vi "Read Signal Message.vi"(6 "timeout ms (25000)":i32=25000, 8 "error in (no error)":errorcluster, 11 "CLI in":refnum<class "CLI.lvclass">) -> (0 "error out":errorcluster, 1 "Message Contents":string, 2 "Message Type":string, 3 "CLI out":refnum<class "CLI.lvclass">)   [LabVIEW 2017, in "CLI.lvclass"]
uses:
  CLI.lvclass
  CLI.lvclass/CLI.ctl
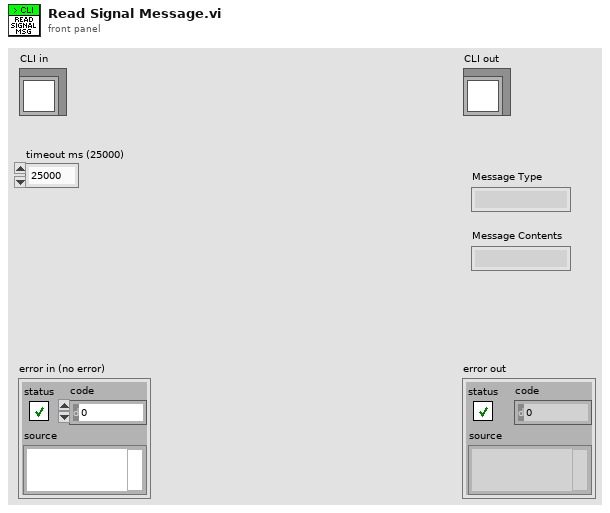
[diagram p1: front panel]
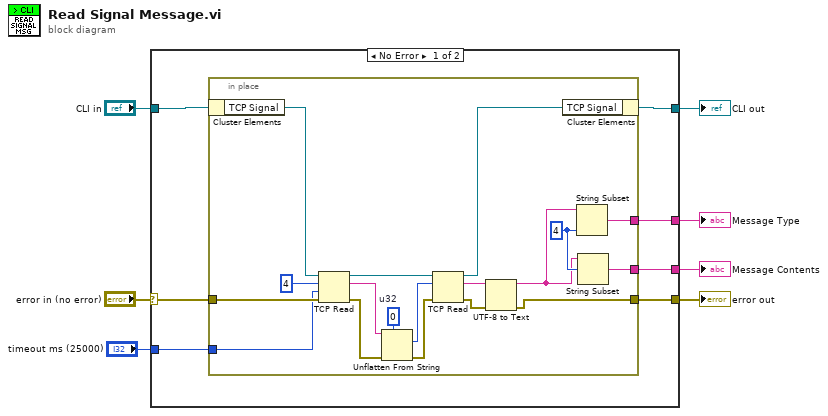
[diagram p0: block diagram]
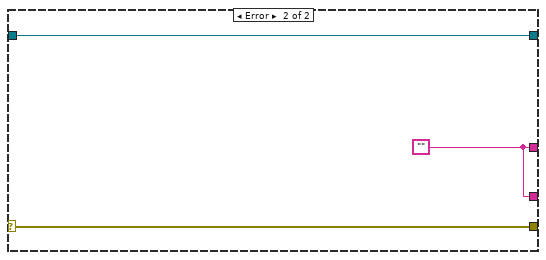
[diagram p2: hidden frame]
diagram:
  n1 = case shown="No Error" "error in (no error)" {
    selector: "error in (no error)" -> [w14 w35]
    tunnel: [w12 w35] -> w6
    tunnel: [w11 w34] -> w4
    tunnel: "CLI in" -> [w13 w34]
    tunnel: [w10 w33] -> w3
    tunnel: [w9 w33] -> w2
    tunnel: "timeout ms (25000)" -> [w8 _]
    frame No Error {
      n2 = in-place {
        in-place-border: w14 -> [w31]
        in-place-border: [w20] -> w12
        in-place-border: [w21] -> w10
        in-place-border: [w19] -> w9
        in-place-border: w8 -> [w15]
        w22 = 4 ("length (rest)")
        w24 = 0  # u32
        n3 = in-place-cluster #1(w13) -> ("TCP Signal"=w32:refnum<k5>)
        n4 = TCP Read(connection ID=w32, bytes to read=4, error in (no error)=w31, 9:w15) -> (connection ID out=w29:refnum<k5>, data out=w25:string, error out=w30:errorcluster)  [unwired: 1 in]
        n5 = Unflatten From String(type=w24, binary string=w25, error in (no error)=w30) -> (value=w23:i32, error out=w26:errorcluster)  [unwired: 2 in, 1 out]
        n6 = TCP Read(connection ID=w29, bytes to read=w23, error in (no error)=w26) -> (connection ID out=w28:refnum<k5>, data out=w18:string, error out=w17:errorcluster)  [unwired: 2 in]
        n7 = UTF-8 to Text(8:w17, 11:w18) -> (0:w20:errorcluster, 3:w16:string)  [unwired: 1 in]
        n8 = in-place-cluster #1("TCP Signal"=w28) -> (w11:refnum<class "CLI.lvclass">)
        n9 = String Subset(string=w16, length (rest)=w22) -> (substring=w21:string)  [unwired: 1 in]
        n10 = String Subset(string=w16, offset (0)=w22) -> (substring=w19:string)  [unwired: 1 in]
      }
    }
    frame Error {
      w33 = ""
    }
  }
  "error out" <- w6
  "CLI out" <- w4
  "Message Type" <- w3
  "Message Contents" <- w2
